vi "LV SCISDK Set Parameter Integer.vi"(8 "error in (no error)":errorcluster, 9 "handle":u64, 10 "value":i32, 11 "Path":string) -> (0 "error out":errorcluster, 1 "handle out":u64, 3 "function return":i32)   [LabVIEW 2021, in "SciSDK_Labview.lvlib"]
doc: "SCISDKLABVIEW_DLL_API int LV_SCISDK_SetParameterInteger(char* Path, int value, void* handle);"
uses:
  SciSDK_Labview.lvlib
  SciSDK_Labview.dll
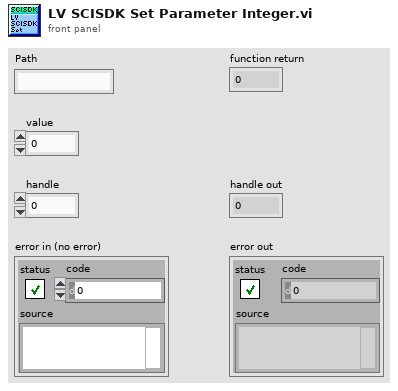
[diagram p1: front panel]
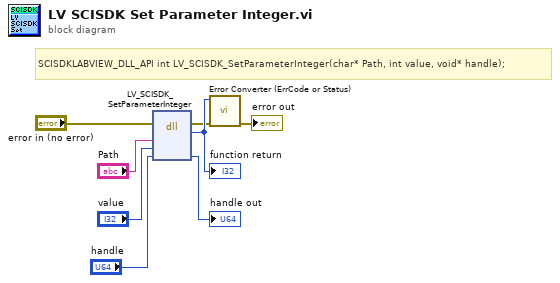
[diagram p0: block diagram]
diagram:
  # "SCISDKLABVIEW_DLL_API int LV_SCISDK_SetParameterInteger(char* Path, int value, void* handle);"
  n1 = dll-call lib="C:/git/scisdk/wrapper/LabView/SciSDK_Labview.*" fn="LV_SCISDK_SetParameterInteger"(error in="error in (no error)", "Path"="Path", "value"="value", "handle"="handle") -> (error out=w2:errorcluster, w8:i32, "handle"=→"handle out":u64)  [unwired: 4 in, 1 out]
  "function return" <- w8
  n2 = call "Error Converter (ErrCode or Status).vi"("error in (no error)"=w2, "error code"=w8) -> ("error out"=→"error out":errorcluster)  [unwired: 9 in]
